vi "PXI_Host_U8_Write_OldMethod_Benchmark.vi"() -> ()   [LabVIEW 2018]
uses:
  <vilib>/addons/FPGA Advanced Session Resources/LVFPGA Adv Session Resources/OpenByNameSubVI.vi
  <vilib>/rvi/interface/common/dynamic/niFpgaEscapeDelimiterAndNull.vi
  <vilib>/Utility/error.llb/Error Cluster From Error Code.vi
  <vilib>/rvi/errors/niLvFpgaAdjustHostInterfaceError.vi
  <vilib>/FPGAPlugInAG/Dynamic/niLvFpga_Close_Dynamic.vi
  <vilib>/addons/FPGA Advanced Session Resources/LVFPGA Adv Session Resources/OpenByName.xnode
  <vilib>/rvi/interface/nirviReadWriteControl/nirviReadWriteControl.xnode
  <vilib>/rvi/interface/nirviCloseFPGA/nirviCloseFPGA.xnode
  NiFpgaLv.dll
  <vilib>/rvi/interface/Simulation/niFpgaSimulationCallBeginRW.vi
  <vilib>/addons/FPGA Advanced Session Resources/LVFPGA Adv Session Resources/LVFPGAAdvSessionResources.lvlib
panel:
  out "error out":errorcluster
  out "Execution time (s)":dbl
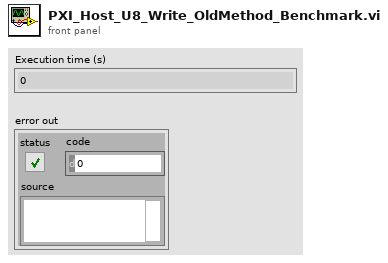
[diagram p1: front panel]
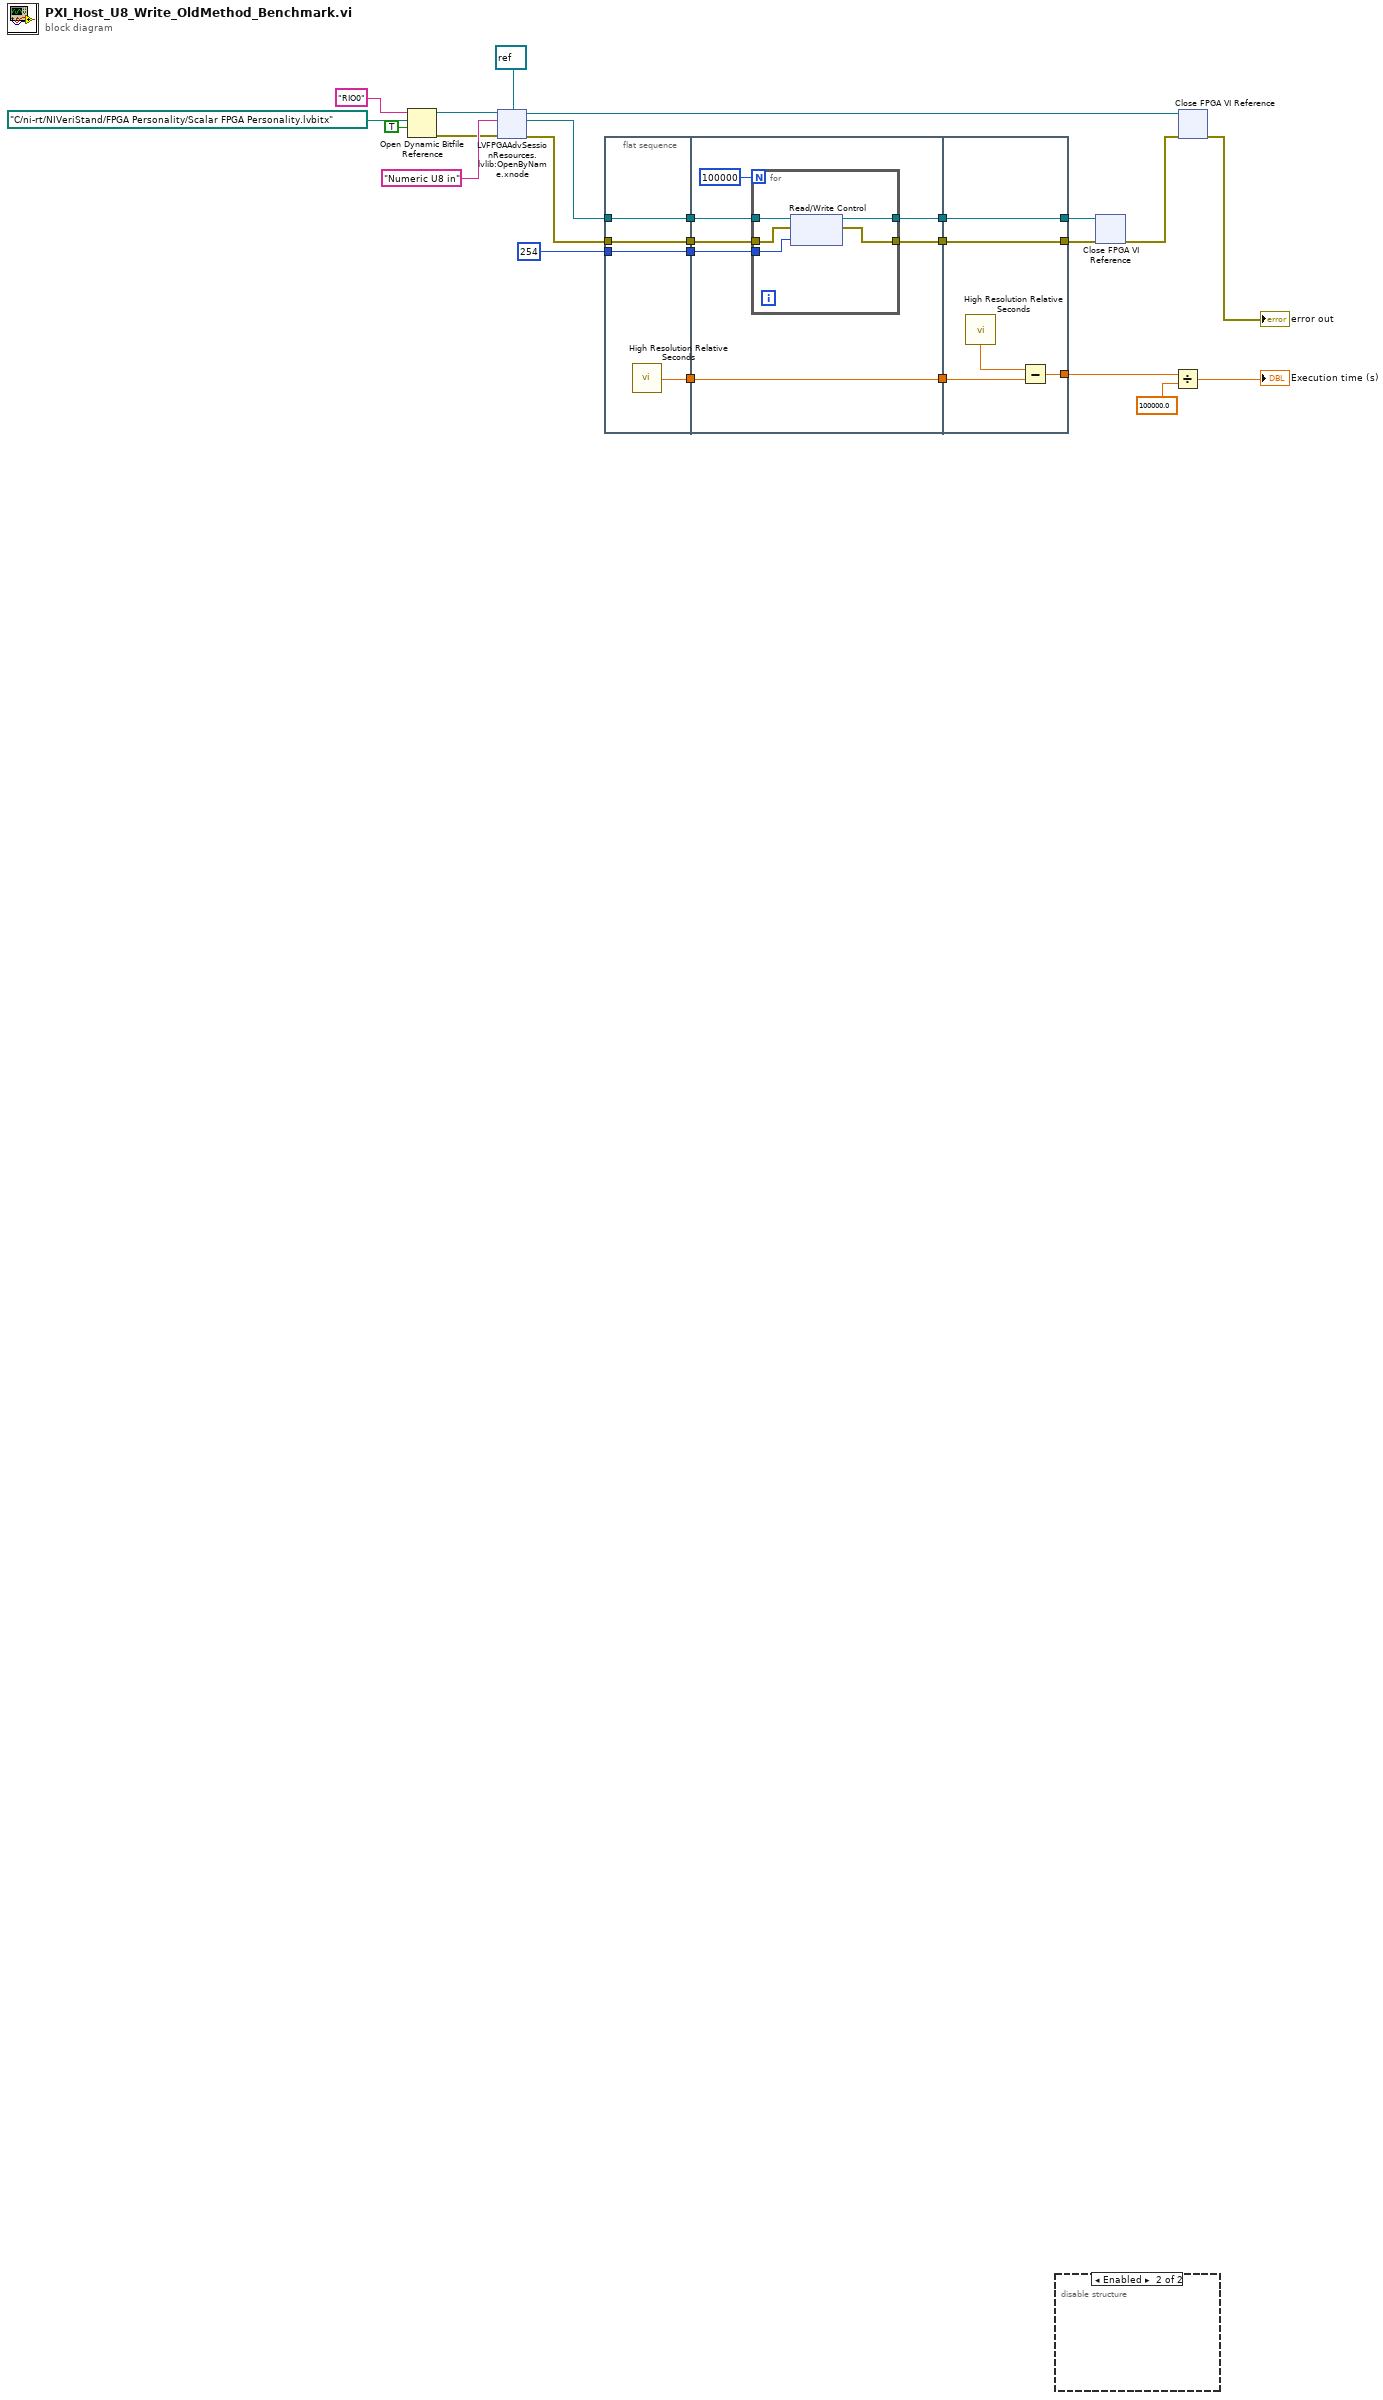
[diagram p0: block diagram]
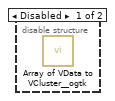
[diagram p2: hidden frame]
diagram:
  n1 = Open Dynamic Bitfile Reference(0:"RIO0" ("Device address"), 1:path "C:/ni-rt/NIVeriStand/FPGA Personality/Scalar FPGA Personality.lvbitx" ("Bitfile path"), 2:TRUE ("Run When Loaded")) -> (5:w13:refnum<k20>, 8:w11:errorcluster)  [unwired: 2 in]
  n2 = xnode "LVFPGAAdvSessionResources.lvlib:OpenByName.xnode"("FPGA VI Reference in"=w13, "Resource name in"="Numeric U8 in", "Single resource reference type in"=refnum<k20> refnum ("Type"), "Error in"=w11) -> ("Single resource reference out"=w9:refnum<k20>, "Error out"=w10:errorcluster, "FPGA VI Reference out"=w4:refnum<k20>)
  n3 = flat-sequence {
    tunnel: [w29] -> w24
    tunnel: w9 -> [w28]
    tunnel: [w28] -> w17
    tunnel: [w27] -> w16
    tunnel: w10 -> [w27]
    tunnel: [w26] -> w2
    tunnel: u8 254 ("Value") -> [w26]
    tunnel: [w35] -> w25
    tunnel: w24 -> [w35]
    tunnel: w17 -> [w34]
    tunnel: w16 -> [w33]
    tunnel: [w32] -> w15
    tunnel: [w31] -> w7
    tunnel: w2 -> [w30]
    tunnel: w25 -> [w45]
    tunnel: [w44] -> w23
    tunnel: w15 -> [w43]
    tunnel: [w43] -> w14
    tunnel: w7 -> [w42]
    tunnel: [w42] -> w6
    frame #0 {
      n4 = call <vilib>:"High Resolution Relative Seconds.vi"() -> ("relative seconds"=w29:dbl)
    }
    frame #1 {
      n5 = for {
        N: 100000 -> [_]
        tunnel: w34 -> [w41]
        tunnel: w33 -> [w40]
        tunnel: [w39] -> w32
        tunnel: [w38] -> w31
        tunnel: w30 -> [w37]
        n6 = xnode "Read/Write Control"("FPGA VI Reference In"=w41, "error in"=w40, "Value"=w37) -> ("FPGA VI Reference Out"=w38:refnum<k20>, "error out"=w39:errorcluster)
      }
    }
    frame #2 {
      n7 = call <vilib>:"High Resolution Relative Seconds.vi"() -> ("relative seconds"=w46:dbl)
      n8 = Subtract(x=w46, y=w45) -> (x-y=w44:dbl)
    }
  }
  n9 = disable-structure shown="Enabled" {
    frame Disabled {
      n10 = call <userlib>:"Array of VData to VCluster__ogtk.vi"() -> ()  [unwired: 10 in, 2 out]
    }
    frame Enabled {
    }
  }
  n11 = xnode "Close FPGA VI Reference"("FPGA VI Reference In"=w6, "error in"=w14) -> ("error out"=w5:errorcluster)
  n12 = Divide(x=w23, y=100000.0) -> (x/y=→"Execution time (s)":dbl)
  n13 = xnode "Close FPGA VI Reference"("FPGA VI Reference In"=w4, "error in"=w5) -> ("error out"=→"error out":errorcluster)
